vi "Add Block Diagram Content.vi"(8 "error in (no error)":errorcluster, 9 "Term Refnum":refnum<vi>, 10 "ModuleLoop":T1, 11 "FPGA Addon Input.lvclass":refnum<class "FPGA Addon Input.lvclass">) -> (0 "error out":errorcluster, 3 "FPGA Addon Input.lvclass":refnum<class "FPGA Addon Input.lvclass">)   [LabVIEW 2015, in "FPGA Addon Input.lvclass"]
uses:
  FPGA Addon Input.lvclass
  Loop/Block Diagram/Module.Refs.ctl
  <vilib>/Utility/miscctls.llb/LVPointTypeDef.ctl
  SubVIs/FPGAAddon.SpecialityInputs.Generate.Parameters.ctl
  Loop/Block Diagram/Block Diagram.lvclass
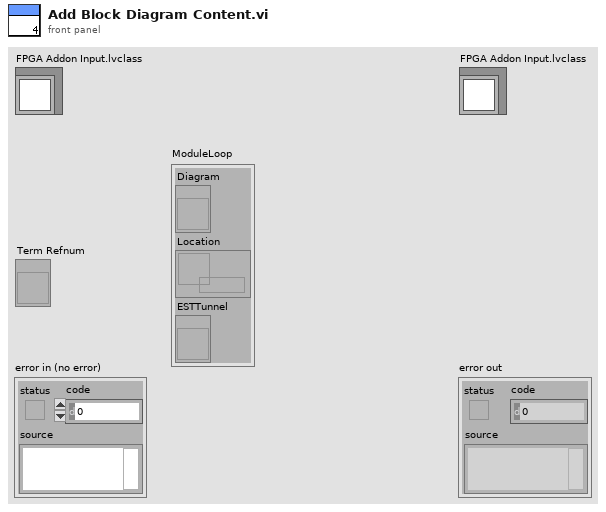
[diagram p1: front panel]
types:
  T1 = typedef "Block Diagram.lvclass/Module.Refs.ctl" = cluster{"Diagram":refnum<vi>, "Location":refnum<data-value>, "ESTTunnel":refnum<vi>}
  T2 = typedef "FPGAAddon.SpecialityInputs.Generate.Parameters.ctl" = cluster{"Parent":refnum<vi>, "subVI path":path, "IO Name":string, "IO Ref":refnum<vi>}
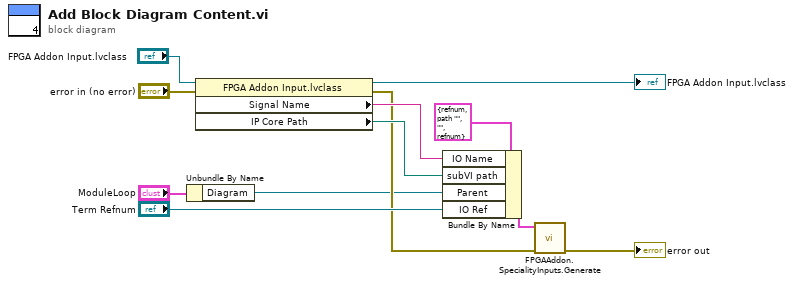
[diagram p0: block diagram]
diagram:
  n1 = Unbundle By Name("ModuleLoop") -> ("Diagram"=w2:refnum<vi>)
  n2 = property class="FPGA Addon Input.lvclass"(reference="FPGA Addon Input.lvclass", error in="error in (no error)") -> (reference out=→"FPGA Addon Input.lvclass":refnum<class "FPGA Addon Input.lvclass">, error out=w4:errorcluster, "Signal Name"=w10:string, "IP Core Path"=w9:path)
  n3 = Bundle By Name(cluster=T2 {"Parent"=refnum, "subVI path"=path "", "IO Name"="", "IO Ref"=refnum} ("Parameters"), "IO Name"=w10, "subVI path"=w9, "Parent"=w2, "IO Ref"="Term Refnum") -> (w11:T2)
  n4 = call "FPGAAddon.SpecialityInputs.Generate.vi"("error in (no error)"=w4, "Parameters"=w11) -> ("error out"=→"error out":errorcluster)  [unwired: 9 in]
